vi "Main Glue UI.vi"() -> ()   [LabVIEW 2017]
uses:
  Potting Application/UI typedefs/Controller Commands.ctl
  Application Utilities/Console Log/Console Log.lvclass
  UI typedefs/Glue Progress States.ctl
  Procedure Classes/Gluing Procedure/Gluing Procedure.lvclass
  Shared Components/Gantry Class/Gantry Class.lvclass
  Shared Components/WorkTable Class/Type Definitions/Worktable_Mode.ctl
  C:/Program Files/National Instruments/LabVIEW 2017/user.lib/aerotech/2010/Bin/Aerotech.A3200.dll
  Program Files/National Instruments/LabVIEW 2017/user.lib/aerotech/2010/Bin/Aerotech.A3200.dll
  Shared Components/Gantry Class/Type Definitions/Virtual Modes.ctl
  UI typedefs/Glue Progress Bar.ctl
panel:
  out "error out":errorcluster
  out "Progress":T1 scale=0.0..7.0
  in  "Comment":string
  out "Console":string
  in  "Add Comment":bool
  in  "Resume Button":bool
  in  "Suspend Button":bool
  in  "Previous Button":bool
  in  "Execute Step":bool
  in  "Manual Control":bool
  in  "Emergency Stop":bool
  in  "ESTOP References":T2
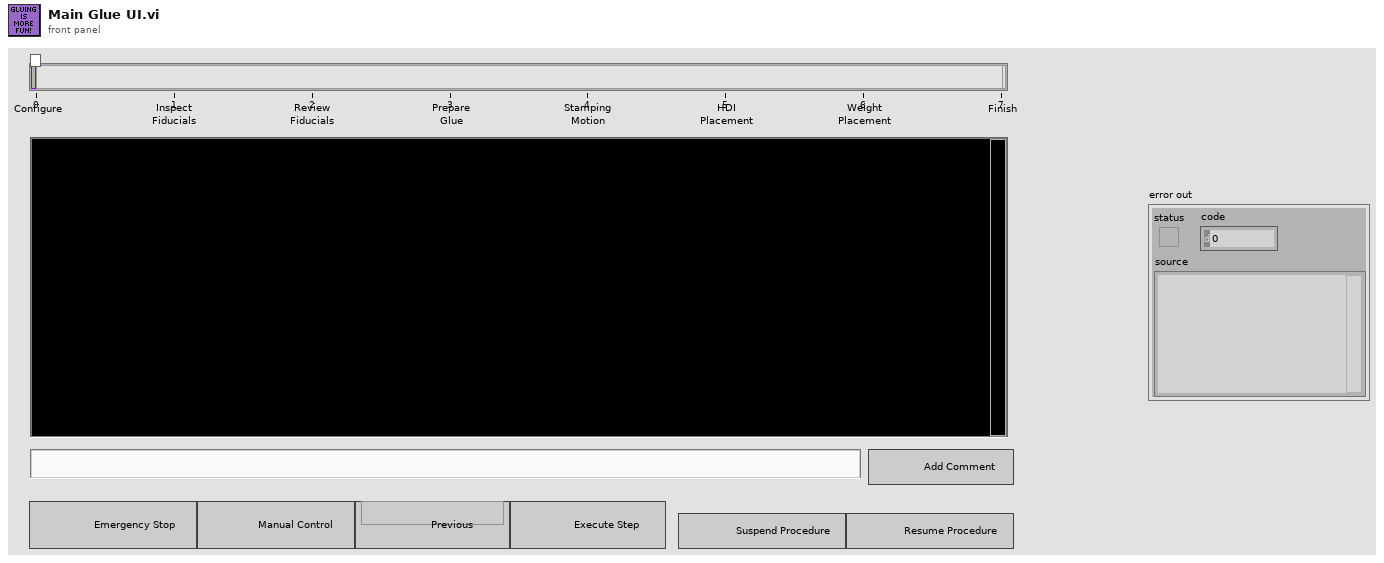
[diagram p1: front panel]
types:
  T1 = typedef "Glue Progress Bar.ctl" = u16
  T2 = cluster{"Aerotech Controller":refnum<k24>, "Manifold Task":refnum<k21>, "Dispenser Task":refnum<k21>}
  T3 = typedef "Glue Progress States.ctl" = enum16{"Configure", "Inspect Fuducials", "Review Fuducials", "Prepare Glue", "Stamping", "HDI Placement", "Weight Placement", "Finish"}
  T4 = typedef "Controller Commands.ctl" = enum16{"Initialize", "Execute Step", "Previous Step", "Add Comment", "Manual Control", "Resume", "Pause", "Emergency Stop"}
  T5 = typedef "Virtual Modes.ctl" = enum16{"Nonvirtual", "Virtual"}
  T6 = cluster{"Aerotech Controller":refnum<k24>, "Dispenser IO Task":refnum<k21>, "Manifold IO Task":refnum<k21>}
  T7 = enum8{"Enabled", "Disabled", "Disabled and Grayed Out"}
  T8 = typedef "Worktable_Mode.ctl" = enum16{"Encapsulation", "Gluing"}
  T9 = enum16{"Left Button", "Center Button", "Right Button", "Window Close"}
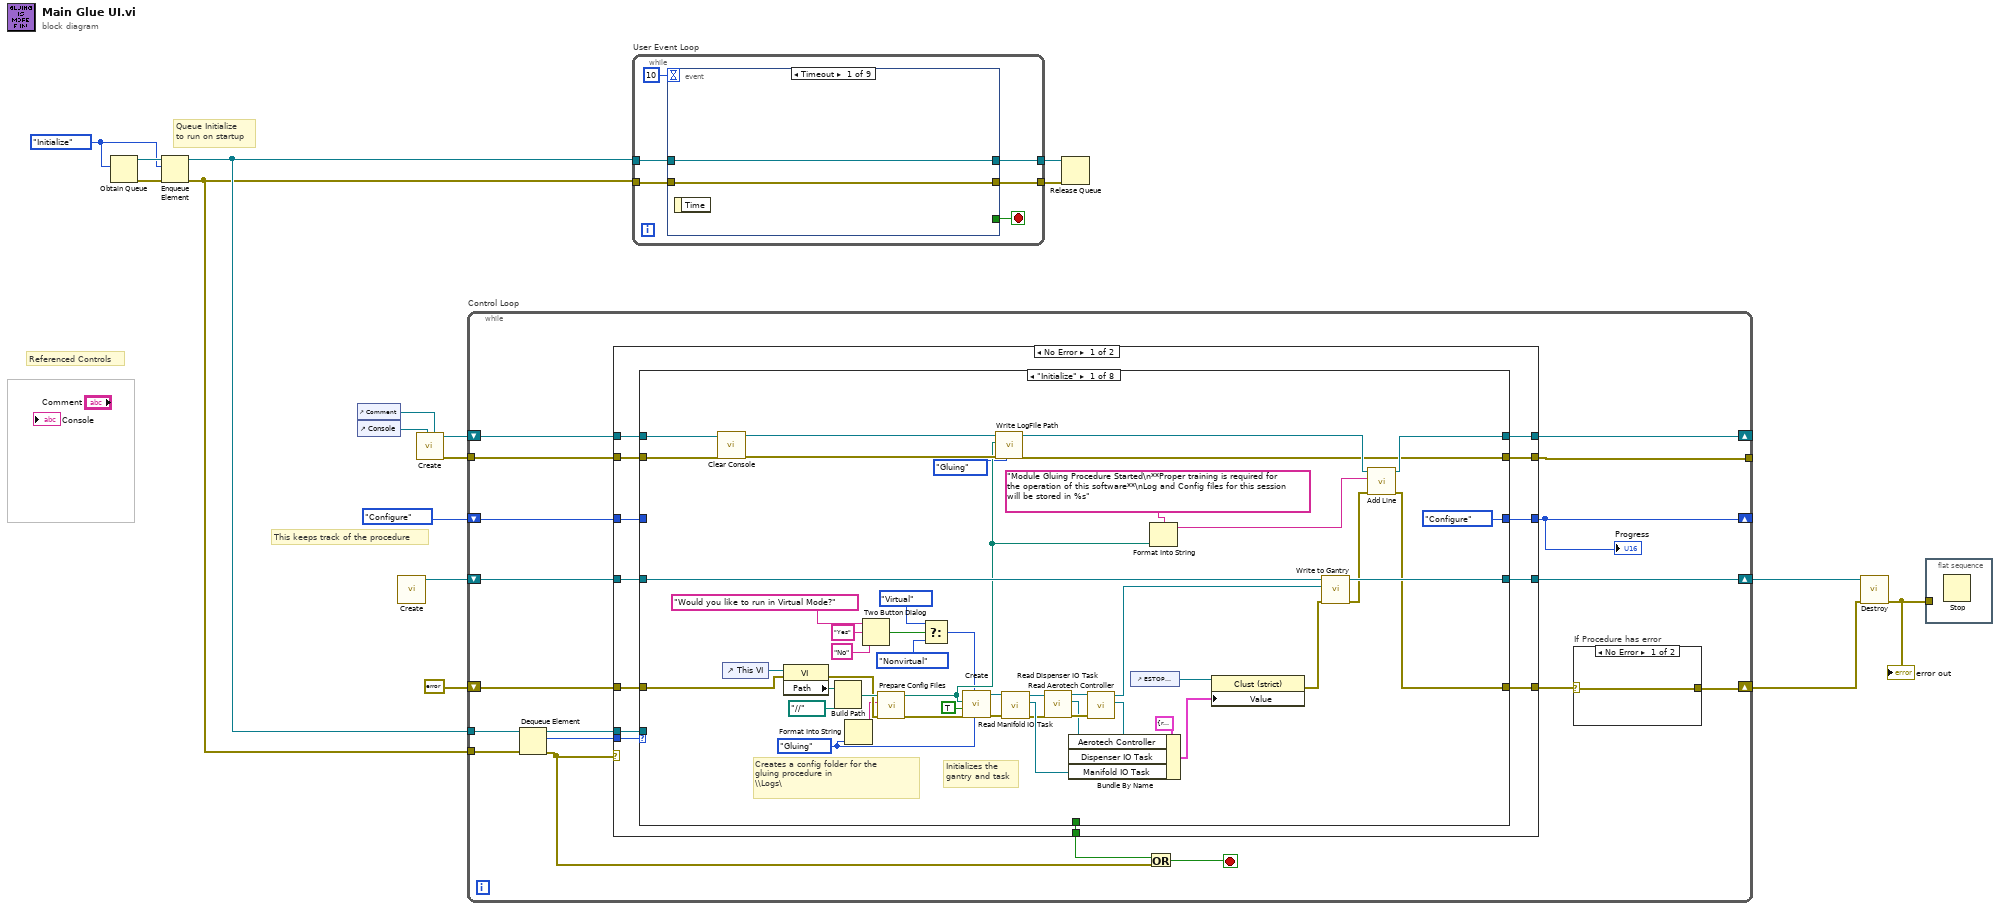
[diagram p0: block diagram]
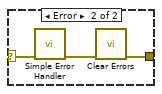
[diagram p2: hidden frame]
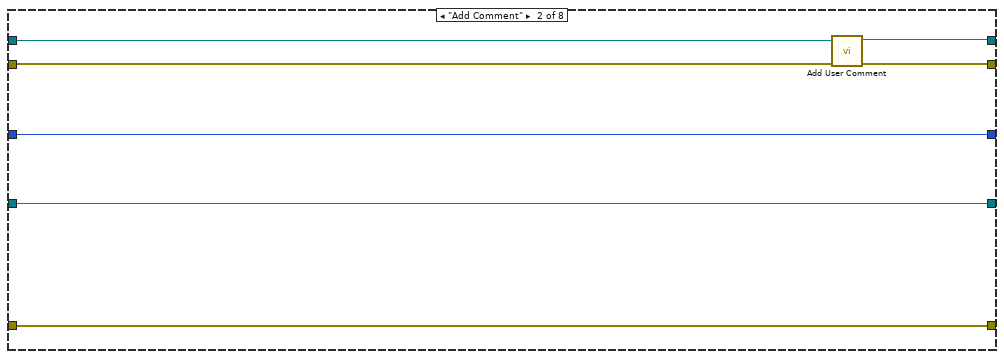
[diagram p3: hidden frame]
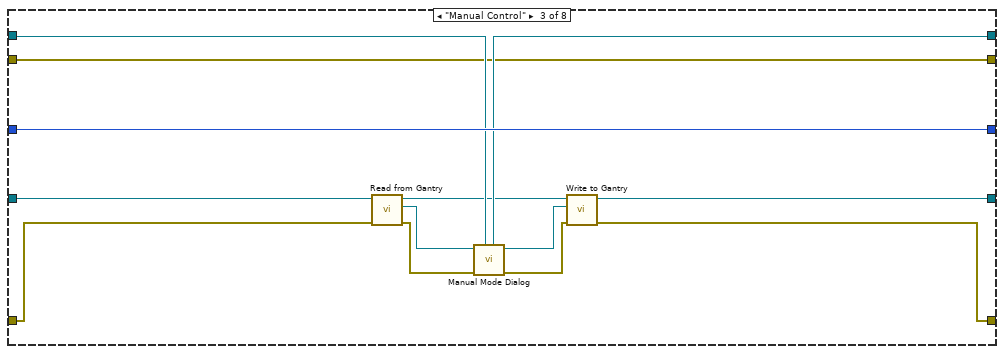
[diagram p4: hidden frame]
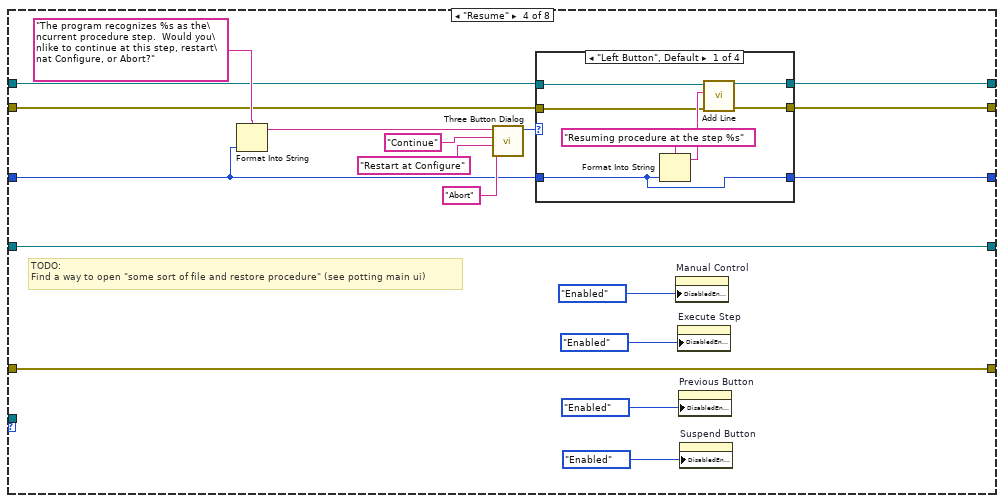
[diagram p5: hidden frame]
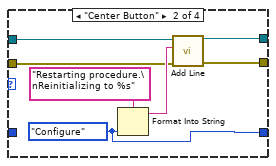
[diagram p6: hidden frame]
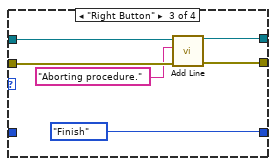
[diagram p7: hidden frame]
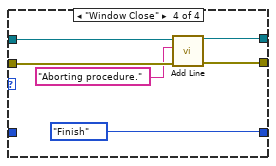
[diagram p8: hidden frame]
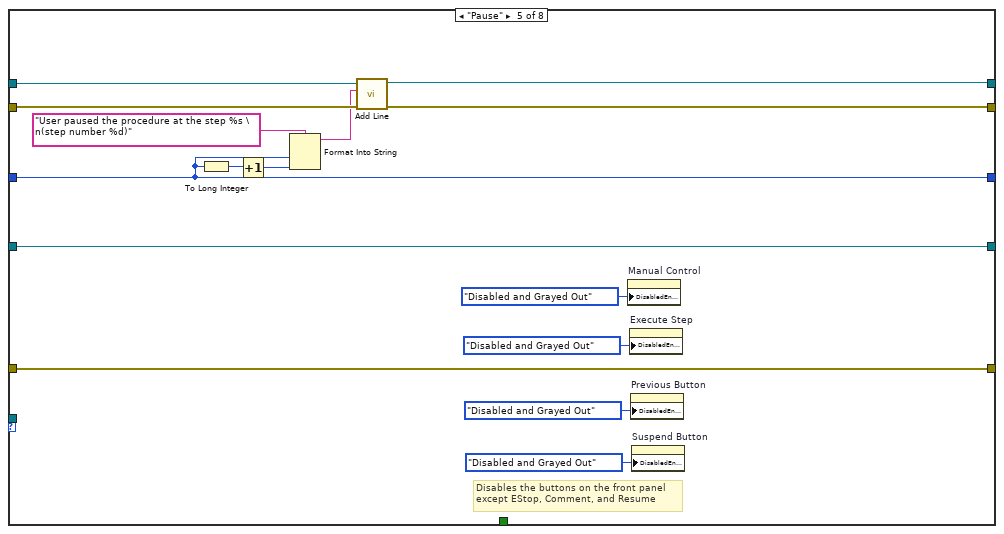
[diagram p9: hidden frame]
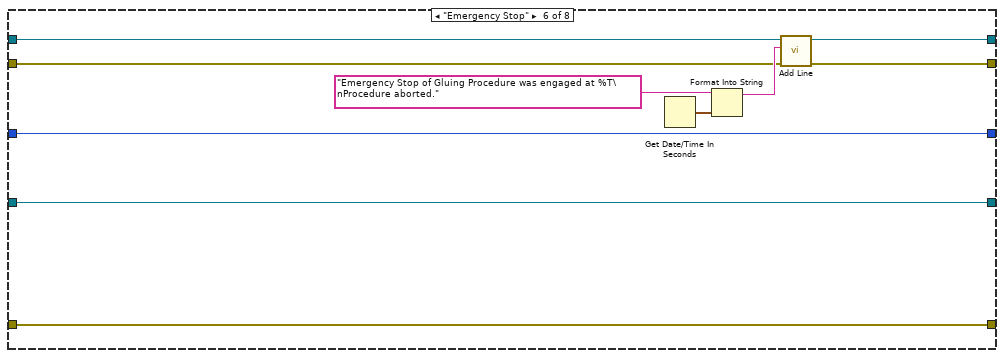
[diagram p10: hidden frame]
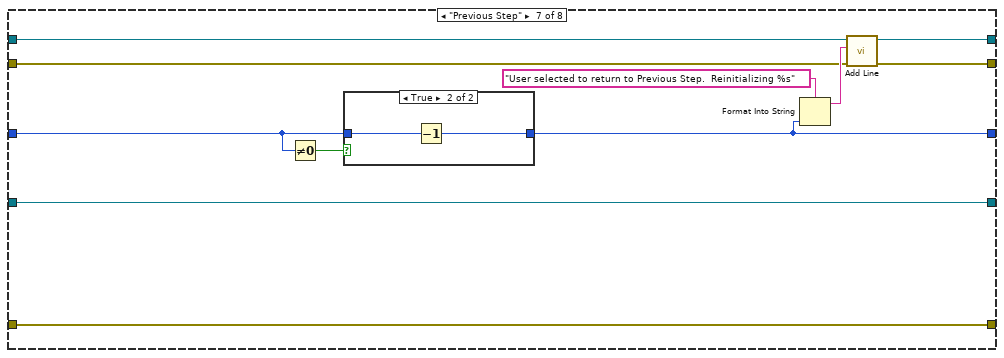
[diagram p11: hidden frame]
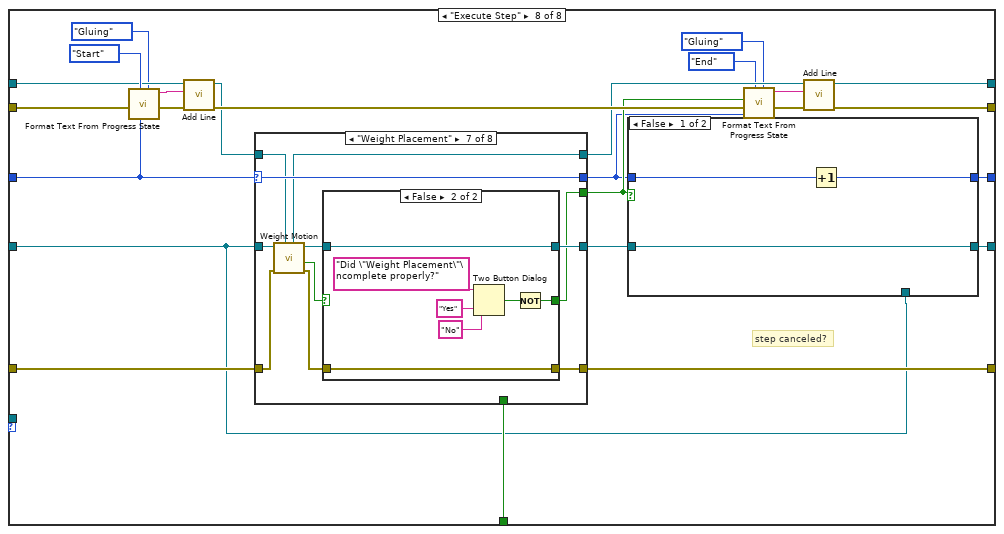
[diagram p13: hidden frame]
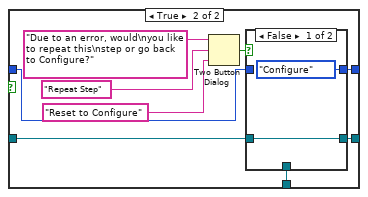
[diagram p14: hidden frame]
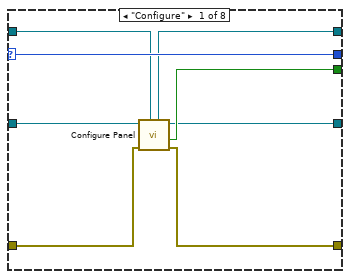
[diagram p16: hidden frame]
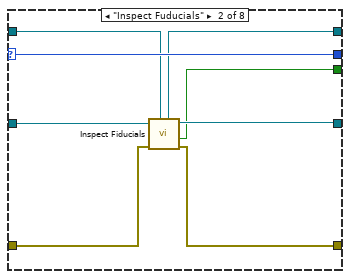
[diagram p17: hidden frame]
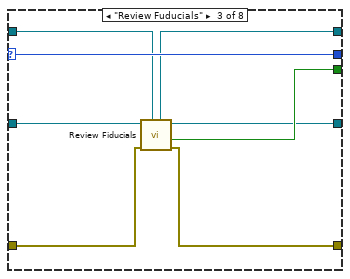
[diagram p18: hidden frame]
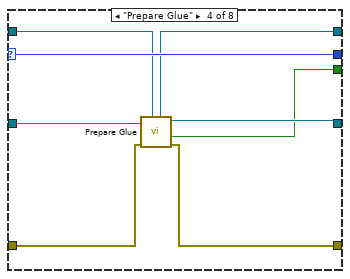
[diagram p19: hidden frame]
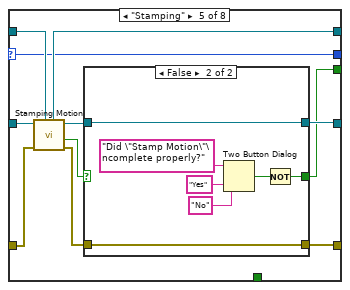
[diagram p20: hidden frame]
diagram:
  w13 = Controller_Commands."Initialize" ("Commands")
  # "This keeps track of the procedure"
  # "Referenced Controls"
  # "Queue Initialize \nto run on startup"
  n1 = Obtain Queue(element data type=w13) -> (queue out=w15:refnum<queue>, error out=w14:errorcluster)  [unwired: 4 in, 1 out]
  n2 = Enqueue Element(queue=w15, element=w13, error in (no error)=w14) -> (queue out=w7:refnum<queue>, error out=w6:errorcluster)  [unwired: 1 in, 1 out]
  n3 = control-ref of="Comment"() -> (w12:refnum<vi>)
  n4 = control-ref of="Console"() -> (w11:refnum<vi>)
  n5 = call "Create.vi"() -> ("Gluing Procedure out"=w1:refnum<class "Gluing Procedure.lvclass">)  [unwired: 10 in, 1 out]
  n6 = call "Create.vi"("Comment"=w12, "Console"=w11) -> ("error out"=w9:errorcluster, "Console Log out"=w10:refnum<class "Console Log.lvclass">)  [unwired: 8 in]
  n7 = while "Control Loop" {
    tunnel: w9 -> [w28]
    shift-right: [w20] -> _
    shift-left: w10 -> [w29]
    shift-right: [w19] -> _
    shift-left: Glue_Progress_States."Configure" ("Enum") -> [w27]
    shift-right: [w22] -> w4
    shift-left: w1 -> [w30]
    shift-right: [w23] -> w2
    shift-left: errorcluster {"status"=FALSE, "code"=0, "source"=""} ("error constant") -> [w31]
    tunnel: w7 -> [w34]
    tunnel: w6 -> [w35]
    tunnel: [w21] -> _
    stop <- w25 stop-if-true
    n8 = Dequeue Element(queue=w34, error in (no error)=w35) -> (queue out=w32:refnum<queue>, element=w33:T4, error out=w26:errorcluster)  [unwired: 1 in, 1 out]
    n9 = case shown="No Error" w26 {
      tunnel: w33 -> [w51 _]
      tunnel: w32 -> [w41 _]
      tunnel: w31 -> [w45 w344]
      tunnel: w30 -> [w46 w345]
      tunnel: w29 -> [w50 w348]
      tunnel: w28 -> [w48 w347]
      tunnel: w27 -> [w52 w346]
      tunnel: [w49 w348] -> w20
      tunnel: [w47 w347] -> w21
      tunnel: [w44 w344] -> w24
      tunnel: [w43 w345] -> w22
      tunnel: [w42 w346] -> w19
      tunnel: [w40 _] -> w18
      frame No Error {
        n10 = case shown="\"Initialize\"" w51 {
          tunnel: w52 -> [_ w106 w119 w127 w170 w188 w198 w215]
          tunnel: w50 -> [w71 w103 w117 w125 w176 w183 w191 w213]
          tunnel: [w67 w102 w118 w134 w172 w185 w195 w210] -> w49
          tunnel: w48 -> [w70 w100 w107 w126 w175 w179 w192 w222]
          tunnel: [w57 w101 w107 w120 w171 w184 w194 w222] -> w47
          tunnel: [Glue_Progress_States."Configure" ("Enum") w106 w119 w135 w170 w188 w190 w221] -> w42
          tunnel: [w73 w105 w108 w137 w178 w187 w197 w217] -> w43
          tunnel: w46 -> [w76 w105 w116 w137 w178 w187 w197 w216]
          tunnel: [w58 w104 w109 w136 w177 w186 w196 w220] -> w44
          tunnel: w45 -> [w98 w104 w110 w136 w177 w186 w196 w223]
          tunnel: w41 -> [_ _ _ _ _ _ _ _]
          tunnel: [_ _ _ _ _ _ _ w219] -> w40
          frame "Initialize" {
            w61 = Worktable_Mode."Gluing" ("Worktable Mode")
            # "Initializes the\ngantry and task"
            # "Creates a config folder for the\ngluing procedure in \n\\\\Logs\\"
            n11 = call "Clear Console.vi"("error in (no error)"=w70, "Console Log in"=w71) -> ("error out"=w68:errorcluster, "Console Log out"=w69:refnum<class "Console Log.lvclass">)  [unwired: 8 in]
            n12 = control-ref of="This VI"() -> (w99:refnum<vi>)
            n13 = property class="VI"(reference=w99, error in=w98) -> (error out=w94:errorcluster, "Path"=w97:path)  [unwired: 1 out]
            n14 = Build Path(base path=w97, name or relative path=path "../../..") -> (appended path=w95:path)
            n15 = Format Into String(w61) -> (resulting string=w60:string)  [unwired: 3 in, 1 out]
            n16 = Two Button Dialog(message="Would you like to run in Virtual Mode?", 1:"No" ("F button name (\"Cancel\")"), 2:"Yes" ("T button name (\"OK\")")) -> (T button?=w56:bool)
            n17 = call "Prepare Config Files.vi"("error in"=w94, "Config Prefix"=w60, "Project Root"=w95) -> ("error out"=w92:errorcluster, "Config Directory"=w63:path)  [unwired: 6 in, 1 out]
            n18 = Select(t=Virtual_Modes."Virtual" ("Virtual Mode"), s=w56, f=Virtual_Modes."Nonvirtual" ("Virtual Mode")) -> (s? t:f=w53:T5)
            n19 = call "Create.vi"(6:w61, "Virtual Mode"=w53, "error in"=w92, "HOME?"=TRUE, "Config Folder"=w63) -> ("error out"=w87:errorcluster, "Gantry out"=w88:refnum<class "Gantry Class.lvclass">)  [unwired: 5 in]
            n20 = call-dynamic "Write LogFile Path.vi"(6:enum16{"Potting", "Gluing"}."Gluing" ("Procedure Type"), "error in"=w68, "Log Filename"=w63, "Console Log in"=w69) -> ("error out"=w57:errorcluster, "Console Log out"=w66:refnum<class "Console Log.lvclass">)  [unwired: 6 in]
            n21 = call-dynamic "Read Manifold IO Task.vi"("error in (no error)"=w87, "Gantry Class in"=w88) -> ("error out"=w84:errorcluster, "Manifold IO Task"=w85:refnum<k21>, "Gantry Class out"=w86:refnum<class "Gantry Class.lvclass">)  [unwired: 7 in]
            n22 = call-dynamic "Read Dispenser IO Task.vi"("error in (no error)"=w84, "Gantry Class in"=w86) -> ("error out"=w82:errorcluster, "Dispenser IO Task"=w79:refnum<k21>, "Gantry Class out"=w83:refnum<class "Gantry Class.lvclass">)  [unwired: 7 in]
            n23 = call-dynamic "Read Aerotech Controller.vi"("error in (no error)"=w82, "Gantry Class in"=w83) -> ("Aerotech Controller"=w81:refnum<k24>, "Gantry Class out"=w75:refnum<class "Gantry Class.lvclass">)  [unwired: 7 in, 1 out]
            n24 = Bundle By Name(cluster=T6 {"Aerotech Controller"=refnum, "Dispenser IO Task"="", "Manifold IO Task"=""} ("input cluster"), "Aerotech Controller"=w81, "Dispenser IO Task"=w79, "Manifold IO Task"=w85) -> (w77:T6)
            n25 = control-ref of="ESTOP References"() -> (w78:refnum<vi>)
            n26 = Format Into String(format string="Module Gluing Procedure Started\n**Proper training is required for the operation of this software**\nLog and Config files for this session will be stored in %s" ("String"), w63) -> (resulting string=w65:string)  [unwired: 2 in, 1 out]
            n27 = property class="Clust (strict)"(reference=w78, "Value"=w77) -> (error out=w74:errorcluster)  [unwired: 1 in, 1 out]
            n28 = call "Write to Gantry.vi"("error in (no error)"=w74, "Gantry"=w75, "Gluing Procedure in"=w76) -> ("error out"=w59:errorcluster, "Gluing Procedure out"=w73:refnum<class "Gluing Procedure.lvclass">)  [unwired: 7 in]
            n29 = call "Add Line.vi"("error in"=w59, "String"=w65, "Console Log in"=w66) -> ("error out"=w58:errorcluster, "Console Log out"=w67:refnum<class "Console Log.lvclass">)  [unwired: 7 in]
          }
          frame "Add Comment" {
            n30 = call "Add User Comment.vi"("error in"=w100, "Console Log in"=w103) -> ("error out"=w101:errorcluster, "Console Log out"=w102:refnum<class "Console Log.lvclass">)  [unwired: 8 in]
          }
          frame "Manual Control" {
            n31 = call "Read from Gantry.vi"("error in (no error)"=w110, "Gluing Procedure in"=w116) -> ("error out"=w113:errorcluster, "Gantry"=w115:refnum<class "Gantry Class.lvclass">, "Gluing Procedure out"=w111:refnum<class "Gluing Procedure.lvclass">)  [unwired: 7 in]
            n32 = call "Manual Mode Dialog.vi"("Console Log in"=w117, "error in"=w113, "Gantry in"=w115) -> ("error out"=w112:errorcluster, "Gantry out"=w114:refnum<class "Gantry Class.lvclass">, "Console Log out"=w118:refnum<class "Console Log.lvclass">)  [unwired: 6 in]
            n33 = call "Write to Gantry.vi"("error in (no error)"=w112, "Gantry"=w114, "Gluing Procedure in"=w111) -> ("error out"=w109:errorcluster, "Gluing Procedure out"=w108:refnum<class "Gluing Procedure.lvclass">)  [unwired: 7 in]
          }
          frame "Resume" {
            # "TODO:\nFind a way to open \"some sort of file and restore procedure\" (see potting main ui)"
            n34 = Format Into String(format string="The program recognizes %s as the\ncurrent procedure step.  Would you\nlike to continue at this step, restart\nat Configure, or Abort?" ("Window Title (\"\")"), w127) -> (resulting string=w131:string)  [unwired: 2 in, 1 out]
            n35 = call <vilib>:"Three Button Dialog.vi"("Right Button Text (\"Cancel\")"="Abort" ("Right Button Text (\"Cancel\")"), "Center Button Text (\"No\")"="Restart at Configure" ("Center Button Text (\"No\")"), "Left Button Text (\"Yes\")"="Continue" ("Left Button Text (\"Yes\")"), "message"=w131) -> ("Which Button?"=w133:T9)  [unwired: 7 in]
            n36 = case shown="\"Left Button\", Default" w133 {
              tunnel: [w144 w148 w156 w162] -> w134
              tunnel: [w143 w149 w157 w163] -> w120
              tunnel: w127 -> [w138 _ _ _]
              tunnel: w126 -> [w140 w146 w154 w160]
              tunnel: w125 -> [w139 w147 w155 w161]
              tunnel: [w138 w145 Glue_Progress_States."Finish" ("Enum") Glue_Progress_States."Finish" ("Enum")] -> w135
              frame "Left Button", Default {
                n37 = Format Into String(format string="Resuming procedure at the step %s", w138) -> (resulting string=w142:string)  [unwired: 2 in, 1 out]
                n38 = call "Add Line.vi"("error in"=w140, "String"=w142, "Console Log in"=w139) -> ("error out"=w143:errorcluster, "Console Log out"=w144:refnum<class "Console Log.lvclass">)  [unwired: 7 in]
              }
              frame "Center Button" {
                w145 = Glue_Progress_States."Configure" ("Enum")
                n39 = Format Into String(format string="Restarting procedure.\nReinitializing to %s", w145) -> (resulting string=w150:string)  [unwired: 2 in, 1 out]
                n40 = call "Add Line.vi"("error in"=w146, "String"=w150, "Console Log in"=w147) -> ("error out"=w149:errorcluster, "Console Log out"=w148:refnum<class "Console Log.lvclass">)  [unwired: 7 in]
              }
              frame "Right Button" {
                n41 = call "Add Line.vi"("error in"=w154, "String"="Aborting procedure." ("format string"), "Console Log in"=w155) -> ("error out"=w157:errorcluster, "Console Log out"=w156:refnum<class "Console Log.lvclass">)  [unwired: 7 in]
              }
              frame "Window Close" {
                n42 = call "Add Line.vi"("error in"=w160, "String"="Aborting procedure." ("format string"), "Console Log in"=w161) -> ("error out"=w163:errorcluster, "Console Log out"=w162:refnum<class "Console Log.lvclass">)  [unwired: 7 in]
              }
            }
            n43 = property on="Manual Control" class="Bool (strict)"("DisabledEnum"=T7."Enabled" ("Disabled")) -> ()  [unwired: 2 in, 2 out]
            n44 = property on="Execute Step" class="Bool (strict)"("DisabledEnum"=T7."Enabled" ("Disabled")) -> ()  [unwired: 2 in, 2 out]
            n45 = property on="Previous Button" class="Bool (strict)"("DisabledEnum"=T7."Enabled" ("Disabled")) -> ()  [unwired: 2 in, 2 out]
            n46 = property on="Suspend Button" class="Bool (strict)"("DisabledEnum"=T7."Enabled" ("Disabled")) -> ()  [unwired: 2 in, 2 out]
          }
          frame "Pause" {
            # "Disables the buttons on the front panel\nexcept EStop, Comment, and Resume"
            n47 = To Long Integer(number=w170) -> (32bit integer=w169:i32)
            n48 = Increment(x=w169) -> (x+1=w168:i32)
            n49 = Format Into String(format string="User paused the procedure at the step %s \n(step number %d)", w170, w168) -> (resulting string=w174:string)  [unwired: 2 in, 1 out]
            n50 = call "Add Line.vi"("error in"=w175, "String"=w174, "Console Log in"=w176) -> ("error out"=w171:errorcluster, "Console Log out"=w172:refnum<class "Console Log.lvclass">)  [unwired: 7 in]
            n51 = property on="Manual Control" class="Bool (strict)"("DisabledEnum"=T7."Disabled and Grayed Out" ("Disabled")) -> ()  [unwired: 2 in, 2 out]
            n52 = property on="Execute Step" class="Bool (strict)"("DisabledEnum"=T7."Disabled and Grayed Out" ("Disabled")) -> ()  [unwired: 2 in, 2 out]
            n53 = property on="Previous Button" class="Bool (strict)"("DisabledEnum"=T7."Disabled and Grayed Out" ("Disabled")) -> ()  [unwired: 2 in, 2 out]
            n54 = property on="Suspend Button" class="Bool (strict)"("DisabledEnum"=T7."Disabled and Grayed Out" ("Disabled")) -> ()  [unwired: 2 in, 2 out]
          }
          frame "Emergency Stop" {
            n55 = Get Date/Time In Seconds() -> (seconds since 1Jan1904=w181:timestamp)
            n56 = Format Into String(format string="Emergency Stop of Gluing Procedure was engaged at %T\nProcedure aborted.", w181) -> (resulting string=w182:string)  [unwired: 2 in, 1 out]
            n57 = call "Add Line.vi"("error in"=w179, "String"=w182, "Console Log in"=w183) -> ("error out"=w184:errorcluster, "Console Log out"=w185:refnum<class "Console Log.lvclass">)  [unwired: 7 in]
          }
          frame "Previous Step" {
            n58 = Not Equal To 0?(x=w198) -> (x != 0?=w199:bool)
            n59 = case shown="True" w199 {
              tunnel: w198 -> [w200 w202]
              tunnel: [w200 w201] -> w190
              frame False {
              }
              frame True {
                n60 = Decrement(x=w202) -> (x-1=w201:T3)
              }
            }
            n61 = Format Into String(format string="User selected to return to Previous Step.  Reinitializing %s", w190) -> (resulting string=w193:string)  [unwired: 2 in, 1 out]
            n62 = call "Add Line.vi"("error in"=w192, "String"=w193, "Console Log in"=w191) -> ("error out"=w194:errorcluster, "Console Log out"=w195:refnum<class "Console Log.lvclass">)  [unwired: 7 in]
          }
          frame "Execute Step" {
            # "step canceled?"
            n63 = call "Format Text From Progress State.vi"("Procedure type"=Worktable_Mode."Gluing", "Glue Procedure Steps"=w215, "Start/End"=enum16{"Start", "End"}."Start") -> ("String"=w212:string)  [unwired: 8 in]
            n64 = call "Add Line.vi"("String"=w212, "Console Log in"=w213) -> ("Console Log out"=w211:refnum<class "Console Log.lvclass">)  [unwired: 8 in, 1 out]
            n65 = case shown="\"Weight Placement\"" w215 {
              selector: w215 -> [w247 w252 w262 w266 w279 w302 w323 w340]
              tunnel: w216 -> [w242 w255 w263 w271 w282 w303 w324 w343]
              tunnel: w223 -> [w241 w249 w257 w267 w278 w299 w320 w337]
              tunnel: w211 -> [w246 w251 w261 w265 w281 w301 w322 w342]
              tunnel: [_ _ _ _ _ _ _ TRUE] -> w219
              tunnel: [w247 w252 w262 w266 w279 w302 w323 w340] -> w205
              tunnel: [w245 w250 w260 w264 w280 w300 w321 w341] -> w208
              tunnel: [w243 w254 w258 w270 w276 w293 w318 w338] -> w218
              tunnel: [w240 w248 w256 w268 w275 w295 w314 w336] -> w220
              tunnel: [w244 w253 w259 w269 w272 w297 w317 w339] -> w206
              frame "Configure" {
                n66 = call "Configure Panel.vi"("Console Log in"=w246, "error in"=w241, "Gluing Procedure in"=w242) -> ("error out"=w240:errorcluster, "Cancel Button status"=w244:bool, "Gluing Procedure out"=w243:refnum<class "Gluing Procedure.lvclass">, "Console Log out"=w245:refnum<class "Console Log.lvclass">)  [unwired: 5 in]
              }
              frame "Inspect Fuducials" {
                n67 = call "Inspect Fiducials.vi"("Console Log in"=w251, "error in"=w249, "Gluing Procedure in"=w255) -> ("error out"=w248:errorcluster, "Step canceled?"=w253:bool, "Gluing Procedure out"=w254:refnum<class "Gluing Procedure.lvclass">, "Console Log out"=w250:refnum<class "Console Log.lvclass">)  [unwired: 5 in]
              }
              frame "Review Fuducials" {
                n68 = call "Review Fiducials.vi"("Console Log in"=w261, "error in"=w257, "Gluing Procedure in"=w263) -> ("error out"=w256:errorcluster, "Step canceled?"=w259:bool, "Gluing Procedure out"=w258:refnum<class "Gluing Procedure.lvclass">, "Console Log out"=w260:refnum<class "Console Log.lvclass">)  [unwired: 5 in]
              }
              frame "Prepare Glue" {
                n69 = call "Prepare Glue.vi"("Console Log in"=w265, "error in"=w267, "Gluing Procedure in"=w271) -> ("error out"=w268:errorcluster, "Step canceled?"=w269:bool, "Gluing Procedure out"=w270:refnum<class "Gluing Procedure.lvclass">, "Console Log out"=w264:refnum<class "Console Log.lvclass">)  [unwired: 5 in]
              }
              frame "Stamping" {
                n70 = call "Stamping Motion.vi"("Console Log in"=w281, "error in"=w278, "Gluing Procedure in"=w282) -> ("error out"=w274:errorcluster, "Step canceled?"=w273:bool, "Gluing Procedure out"=w277:refnum<class "Gluing Procedure.lvclass">, "Console Log out"=w280:refnum<class "Console Log.lvclass">)  [unwired: 5 in]
                n71 = case shown="False" w273 {
                  selector: w273 -> [w285 _]
                  tunnel: [w285 w289] -> w272
                  tunnel: w274 -> [w283 w287]
                  tunnel: [w283 w287] -> w275
                  tunnel: w277 -> [w284 w286]
                  tunnel: [w284 w286] -> w276
                  frame True {
                  }
                  frame False {
                    n72 = Two Button Dialog(message="Did \"Stamp Motion\"\ncomplete properly?", 1:"No" ("F button name (\"Cancel\")"), 2:"Yes" ("T button name (\"OK\")")) -> (T button?=w288:bool)
                    n73 = Not(x=w288) -> (.not. x?=w289:bool)
                  }
                }
              }
              frame "HDI Placement" {
                n74 = call "HDI Placement motion.vi"("Console Log in"=w301, "error in"=w299, "Gluing Procedure in"=w303) -> ("error out"=w296:errorcluster, "Step canceled?"=w298:bool, "Gluing Procedure out"=w294:refnum<class "Gluing Procedure.lvclass">, "Console Log out"=w300:refnum<class "Console Log.lvclass">)  [unwired: 5 in]
                n75 = case shown="False" w298 {
                  selector: w298 -> [w306 _]
                  tunnel: [w306 w310] -> w297
                  tunnel: w296 -> [w304 w308]
                  tunnel: [w304 w308] -> w295
                  tunnel: w294 -> [w305 w307]
                  tunnel: [w305 w307] -> w293
                  frame True {
                  }
                  frame False {
                    n76 = Two Button Dialog(message="Did \"HDI Placement\"\ncomplete properly?", 1:"No" ("F button name (\"Cancel\")"), 2:"Yes" ("T button name (\"OK\")")) -> (T button?=w309:bool)
                    n77 = Not(x=w309) -> (.not. x?=w310:bool)
                  }
                }
              }
              frame "Weight Placement" {
                n78 = call "Weight Motion.vi"("Console Log in"=w322, "error in"=w320, "Gluing Procedure in"=w324) -> ("error out"=w315:errorcluster, "Step canceled?"=w316:bool, "Gluing Procedure out"=w319:refnum<class "Gluing Procedure.lvclass">, "Console Log out"=w321:refnum<class "Console Log.lvclass">)  [unwired: 5 in]
                n79 = case shown="False" w316 {
                  selector: w316 -> [w327 _]
                  tunnel: [w327 w331] -> w317
                  tunnel: w315 -> [w325 w329]
                  tunnel: [w325 w329] -> w314
                  tunnel: w319 -> [w326 w328]
                  tunnel: [w326 w328] -> w318
                  frame True {
                  }
                  frame False {
                    n80 = Two Button Dialog(message="Did \"Weight Placement\"\ncomplete properly?", 1:"No" ("F button name (\"Cancel\")"), 2:"Yes" ("T button name (\"OK\")")) -> (T button?=w330:bool)
                    n81 = Not(x=w330) -> (.not. x?=w331:bool)
                  }
                }
              }
              frame "Finish" {
                n82 = call "Write Log Summary Dialog.vi"("Console Log in"=w342, "error in"=w337, "Gluing Procedure in"=w343) -> ("error out"=w336:errorcluster, "Step canceled?"=w339:bool, "Gluing Procedure out"=w338:refnum<class "Gluing Procedure.lvclass">, "Console Log out"=w341:refnum<class "Console Log.lvclass">)  [unwired: 5 in]
              }
            }
            n83 = case shown="False" w206 {
              tunnel: w205 -> [w226 w231]
              tunnel: [w225 w230] -> w221
              tunnel: w218 -> [w224 w229]
              tunnel: [w224 w228] -> w217
              tunnel: w216 -> [_ w227]
              frame False {
                n84 = Increment(x=w226) -> (x+1=w225:T3)
              }
              frame True {
                n85 = Two Button Dialog(message="Due to an error, would\nyou like to repeat this\nstep or go back to Configure?", 1:"Reset to Configure" ("F button name (\"Cancel\")"), 2:"Repeat Step" ("T button name (\"OK\")")) -> (T button?=w235:bool)
                n86 = case shown="False" w235 {
                  tunnel: w231 -> [_ w239]
                  tunnel: [Glue_Progress_States."Configure" ("Enum") w239] -> w230
                  tunnel: w229 -> [w236 _]
                  tunnel: [w236 w238] -> w228
                  tunnel: w227 -> [_ w238]
                  frame False {
                  }
                  frame True {
                  }
                }
              }
            }
            n87 = call "Format Text From Progress State.vi"("Procedure type"=Worktable_Mode."Gluing", "Glue Procedure Steps"=w205, "Start/End"=enum16{"Start", "End"}."End", "Canceled"=w206) -> ("String"=w209:string)  [unwired: 7 in]
            n88 = call "Add Line.vi"("String"=w209, "Console Log in"=w208) -> ("Console Log out"=w210:refnum<class "Console Log.lvclass">)  [unwired: 8 in, 1 out]
          }
        }
      }
      frame Error {
      }
    }
    "Progress" <- w19
    n89 = Or(x=w18, y=w26) -> (x .or. y?=w25:bool)
    n90 = case "If Procedure has error" shown="No Error" w24 {
      selector: w24 -> [w36 w39]
      tunnel: [w36 w38] -> w23
      frame No Error {
      }
      frame Error {
        n91 = call <vilib>:"Simple Error Handler.vi"("error in (no error)"=w39) -> ("error out"=w37:errorcluster)  [unwired: 4 in, 4 out]
        n92 = call <vilib>:"Clear Errors.vi"("error in (no error)"=w37) -> ("error out"=w38:errorcluster)  [unwired: 5 in, 1 out]
      }
    }
  }
  n93 = while "User Event Loop" {
    tunnel: w7 -> [w349]
    tunnel: [w352] -> w17
    tunnel: w6 -> [w351]
    tunnel: [w350] -> w16
    stop <- w353 stop-if-true
    n94 = event shown="[0] Timeout" {
      selector: _ -> [_ _ _ _ _ _ _ _ _]
      dyn-events: _ -> [_ _ _ _ _ _ _ _ _]
      timeout: 10 -> [_ _ _ _ _ _ _ _ _]
      tunnel: [_ _ _ _ _ _ _ w387 _] -> w353
      tunnel: w349 -> [w356 w359 w363 w369 w371 w377 w382 w386 w393]
      tunnel: [w356 w359 w362 w366 w373 w379 w384 w386 w394] -> w352
      tunnel: w351 -> [w355 w358 w361 w368 w370 w376 w381 w385 w396]
      tunnel: [w355 w358 w360 w367 w372 w378 w380 w385 w395] -> w350
      event Timeout {
        n95 = event-data() -> ()  [unwired: 1 in, 1 out]
      }
      event "Emergency Stop": Mouse Up {
        n96 = event-data() -> ()  [unwired: 1 in, 1 out]
        n97 = call "Emergency Stop.vi"("ESTOP References"="ESTOP References") -> ()
      }
      event "Manual Control": Mouse Up {
        n98 = event-data() -> ()  [unwired: 1 in, 1 out]
        n99 = Enqueue Element(queue=w363, element=Controller_Commands."Manual Control", error in (no error)=w361) -> (queue out=w362:refnum<queue>, error out=w360:errorcluster)  [unwired: 1 in, 1 out]
      }
      event "Execute Step": Mouse Up {
        n100 = event-data() -> ()  [unwired: 1 in, 1 out]
        n101 = Enqueue Element(queue=w369, element=Controller_Commands."Execute Step", error in (no error)=w368) -> (queue out=w366:refnum<queue>, error out=w367:errorcluster)  [unwired: 1 in, 1 out]
      }
      event "Previous Button": Mouse Up {
        n102 = event-data() -> ()  [unwired: 1 in, 1 out]
        n103 = Enqueue Element(queue=w371, element=Controller_Commands."Previous Step", error in (no error)=w370) -> (queue out=w373:refnum<queue>, error out=w372:errorcluster)  [unwired: 1 in, 1 out]
      }
      event "Suspend Button": Mouse Up {
        n104 = event-data() -> ()  [unwired: 1 in, 1 out]
        n105 = Enqueue Element(queue=w377, element=Controller_Commands."Pause", error in (no error)=w376) -> (queue out=w379:refnum<queue>, error out=w378:errorcluster)  [unwired: 1 in, 1 out]
      }
      event "Resume Button": Mouse Up {
        n106 = event-data() -> ()  [unwired: 1 in, 1 out]
        n107 = Enqueue Element(queue=w382, element=Controller_Commands."Resume", error in (no error)=w381) -> (queue out=w384:refnum<queue>, error out=w380:errorcluster)  [unwired: 1 in, 1 out]
      }
      event Panel Close? {
        n108 = event-data() -> ()  [unwired: 1 in, 1 out]
        n109 = Two Button Dialog(message="Are you sure you want to quit?", 1:"Return" ("F button name (\"Cancel\")"), 2:"Quit" ("T button name (\"OK\")")) -> (T button?=w387:bool)
        n110 = event-data("Discard?"=TRUE) -> ()  [unwired: 1 in, 1 out]
      }
      event "Add Comment": Mouse Up {
        n111 = event-data() -> ()  [unwired: 1 in, 1 out]
        n112 = Enqueue Element(queue=w393, element=Controller_Commands."Add Comment", error in (no error)=w396) -> (queue out=w394:refnum<queue>, error out=w395:errorcluster)  [unwired: 1 in, 1 out]
      }
    }
  }
  n113 = Release Queue(queue=w17, error in (no error)=w16) -> ()  [unwired: 1 in, 3 out]
  n114 = call "Destroy.vi"("error in"=w2, "Gluing Procedure in"=w4) -> ("error out"=w3:errorcluster)  [unwired: 9 in]
  "error out" <- w3
  n115 = flat-sequence {
    tunnel: w3 -> [_]
    frame #0 {
      n116 = Stop() -> ()  [unwired: 1 in]
    }
  }
